vi "DATA LOG.vi"() -> ()   [LabVIEW 2023]
panel:
  out "OP 30 SCAN STATUS":bool
  out "OP 20 SCAN STATUS":bool
  out "OP 10 SCAN STATUS":bool
  in  "test barcode":string
  out "scan op 30":bool
  in  "byte to string":string
  in  "string to bye array":u8[](array[numeric])
  out "scan op 60":bool
  out "scan op 40":bool
  in  "op 60":i32=1
  in  "op 40":i32=1
  in  "op 30":i32=2
  out "3":bool
  out "2":bool
  out "1":bool
  out "ST 4 STRING 3":string
  out "ST 3 STRING 2":string
  out "OP30 ST 2 STRING":string
  out "DATA LOG RESET 4":bool
  out "DATA LOG RESET 3":bool
  out "DATA LOG RESET 2":bool
  out "OP 10 DATA LOG RESULT":bool
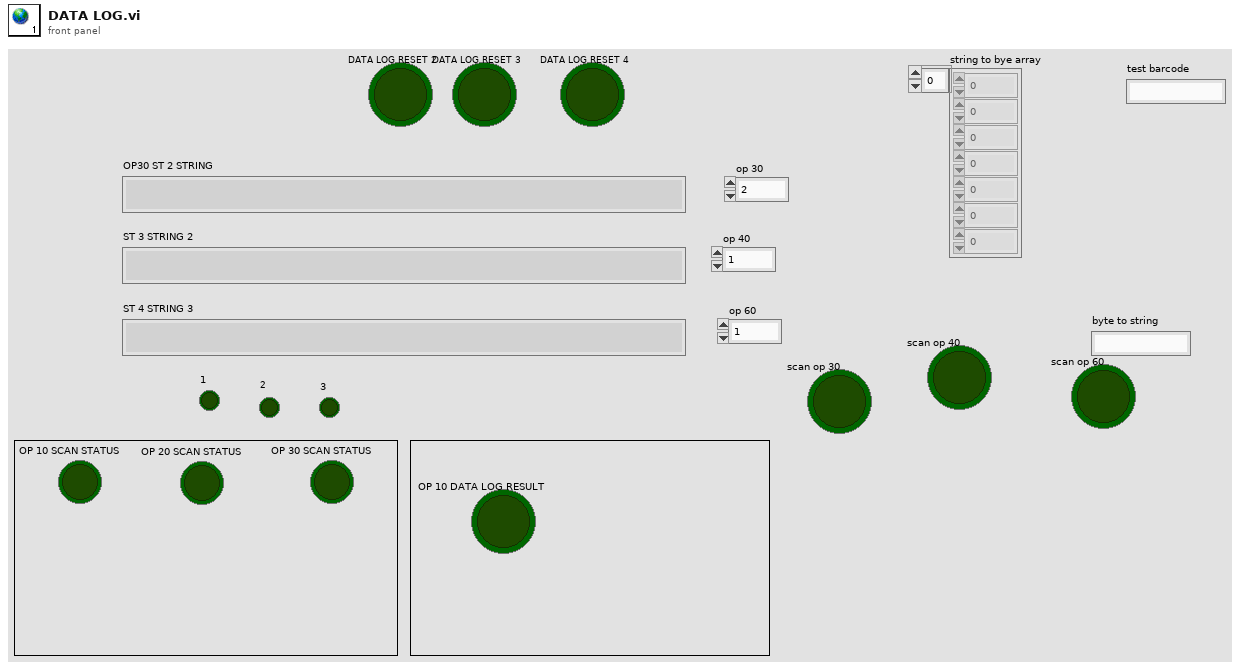
[diagram p1: front panel]
diagram:
